vi "NMEA serial.vi"() -> ()   [LabVIEW 2016, in "AIRMAR WeatherCaster.lvlib"]
uses:
  AIRMAR WeatherCaster.lvlib
  NMEA_WIMDA-data.ctl
  NMEA_GPRMC-data.ctl
  NMEA_LatitudeDirection.ctl
  NMEA_LongitudeDirection.ctl
  <vilib>/Utility/miscctls.llb/LVPointTypeDef.ctl
  <vilib>/Instr/_visa.llb/VISA Configure Serial Port (Instr).vi
panel:
  out "$GPRMC-message_OUT":T1={"TimeStamp"=timestamp(0 s since 1904-01-01), "Validity"=FALSE, "Latitude"=0.0, "Latitude-Direction"=enum."North", "Longitude"=0.0, "Longitude-Direction"=enum."East", "Speed in knots"=0.0, "True course"=0.0, "Date Stamp"=timestamp(0 s since 1904-01-01), "Magnetic Variation (East/West)"=0.0} {"Magnetic Variation (East/West)" format="%.02f [deg]"; "Date Stamp" format="%<%x>T"; "True course" format="%.02f [deg]"; "Speed in knots" format="%.02f [kts]"; "Longitude" format="%0.4f [long]"; "Latitude" format="%.04f [lat]"; "TimeStamp" format="%<%.2X>T"}
  out "风向_真角":dbl caption="风向"
  out "风速_m/s":dbl caption="风速"
  out "风速_节":dbl caption="风速"
  out "气温_摄氏度":dbl caption="气温"
  out "气压_bars":dbl caption="气压"
  out "气压_英寸汞柱":dbl caption="气压"
  out "匹配语句":string
  out "$WIMDA-message_OUT":T4
  in  "串口打开":bool
  out "RAW DATA":string
  in  "baud rate (9600)":u32(ring)=4800 caption="波特率" items=["1200"=1200, "2400"=2400, "4800"=4800, "9600"=9600, "38400"=38400, "115200"=115200]
  in  "VISA resource name":refnum<visa-resource-name> caption="串口"
  # "°"
  # "m/s"
  # "节"
  # "℃"
  # "bars"
  # "英寸汞柱"
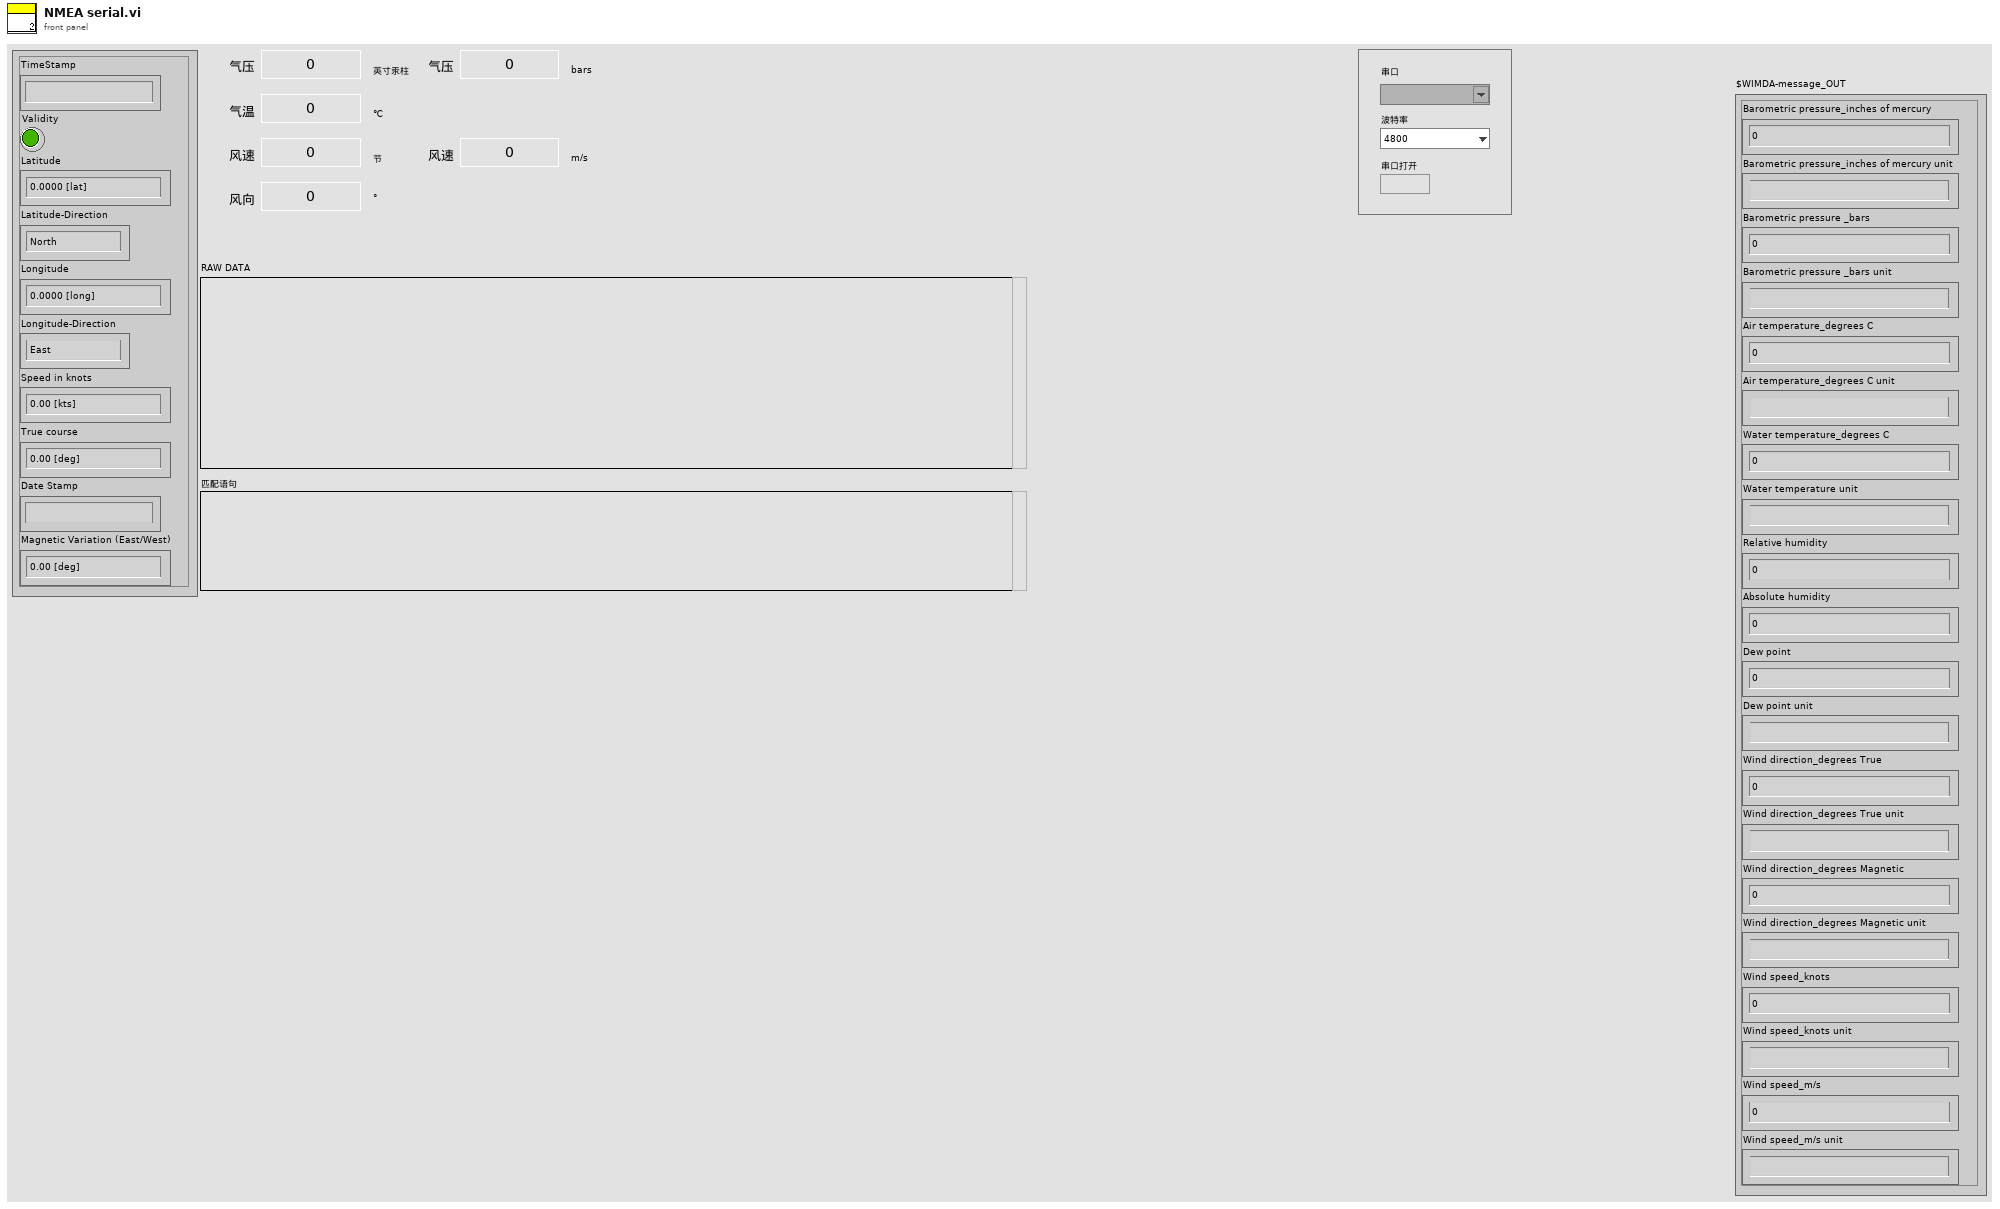
[diagram p1: front panel]
types:
  T1 = typedef "AIRMAR WeatherCaster.lvlib/NMEA_GPRMC-data.ctl" = cluster{"TimeStamp":timestamp, "Validity":bool, "Latitude":dbl, "Latitude-Direction":T2, "Longitude":dbl, "Longitude-Direction":T3, "Speed in knots":dbl, "True course":dbl, "Date Stamp":timestamp, "Magnetic Variation (East/West)":dbl}
  T2 = typedef "AIRMAR WeatherCaster.lvlib/NMEA_LatitudeDirection.ctl" = enum16{"", "North", "South"}
  T3 = typedef "AIRMAR WeatherCaster.lvlib/NMEA_LongitudeDirection.ctl" = enum16{"", "East", "West"}
  T4 = typedef "AIRMAR WeatherCaster.lvlib/NMEA_WIMDA-data.ctl" = cluster{"Barometric pressure_inches of mercury":dbl, "Barometric pressure_inches of mercury unit":string, "Barometric pressure _bars":dbl, "Barometric pressure _bars unit":string, "Air temperature_degrees C":dbl, "Air temperature_degrees C unit":string, "Water temperature_degrees C":dbl, "Water temperature unit":string, "Relative humidity":dbl, "Absolute humidity":dbl, "Dew point":dbl, "Dew point unit":string, "Wind direction_degrees True":dbl, "Wind direction_degrees True unit":string, "Wind direction_degrees Magnetic":dbl, "Wind direction_degrees Magnetic unit":string, "Wind speed_knots":dbl, "Wind speed_knots unit":string, "Wind speed_m/s":dbl, "Wind speed_m/s unit":string}
  T5 = typedef "LVPointTypeDef.ctl" = cluster{"Horizontal":i16, "Vertical":i16}
  T6 = typedef "LVDateTimeRec.ctl" = cluster{"秒数的小数部分":dbl, "秒":i32, "分":i32, "时":i32, "日":i32, "月":i32, "年":i32, "天数（周）":i32, "天数（年）":i32, "DST":i32}
  T7 = enum8{"Enabled", "Disabled", "Disabled and Grayed Out"}
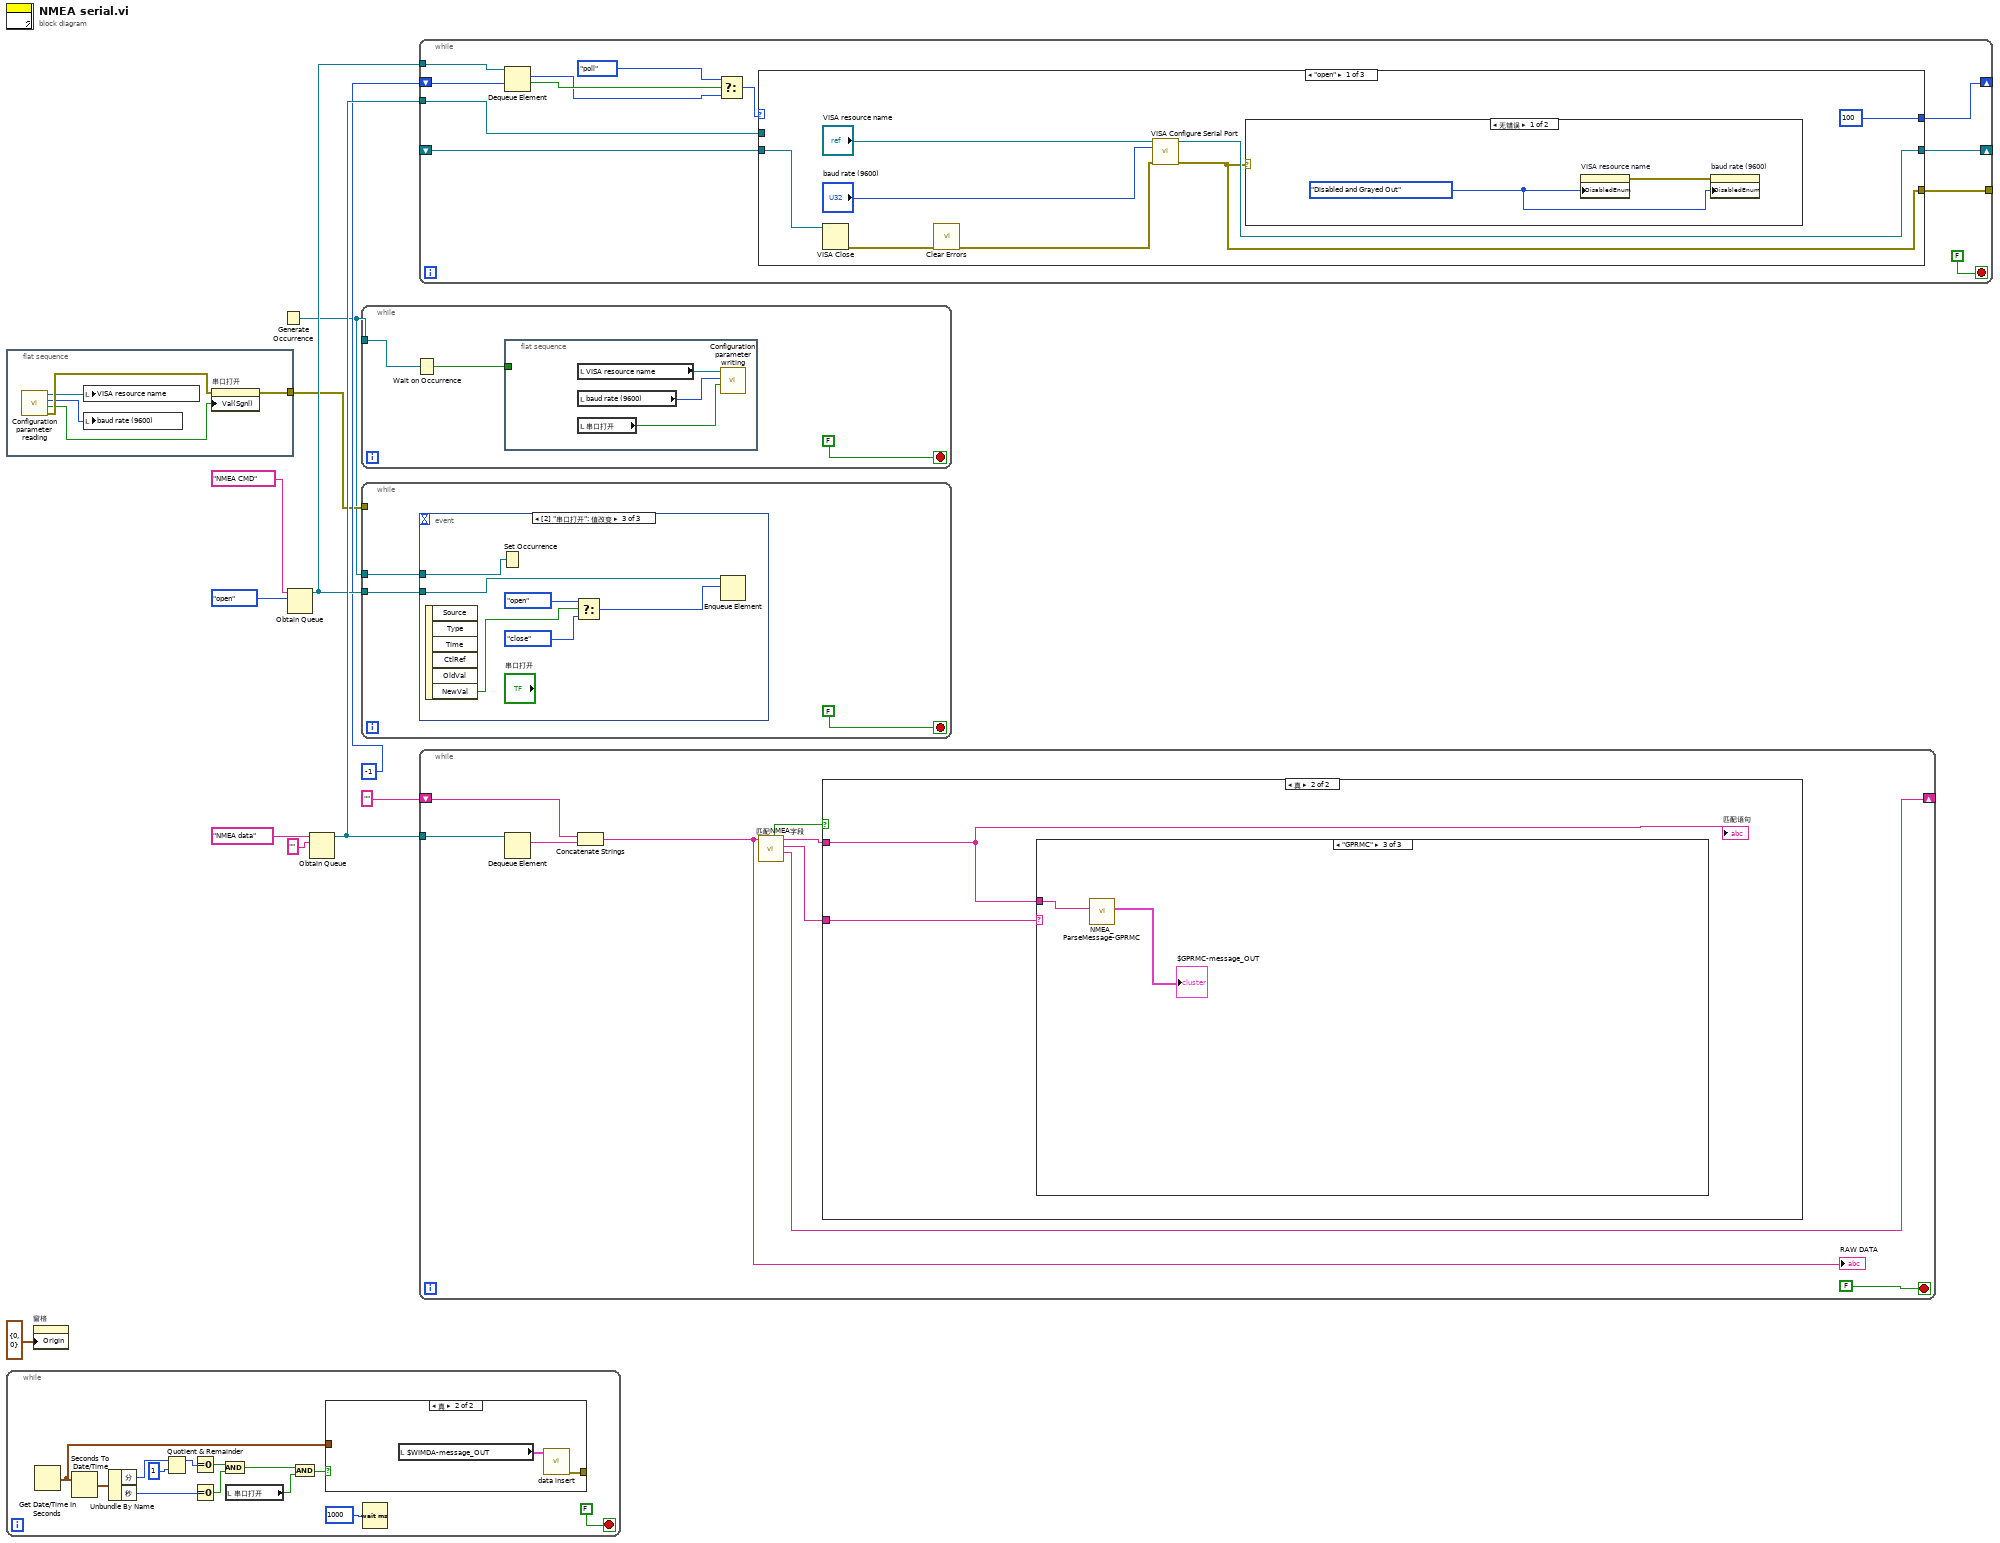
[diagram p0: block diagram]
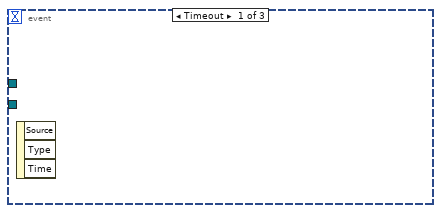
[diagram p3: hidden frame]
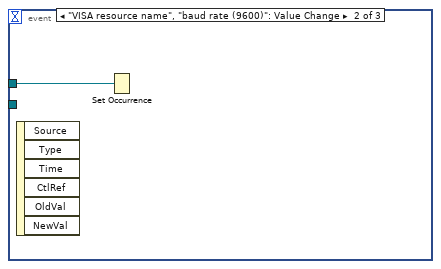
[diagram p4: hidden frame]
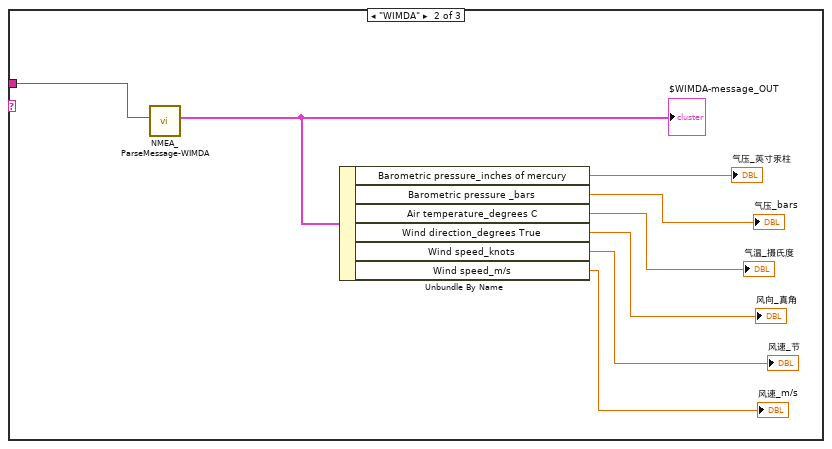
[diagram p7: hidden frame]
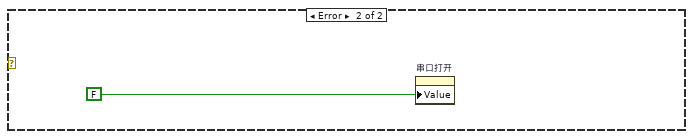
[diagram p8: hidden frame]
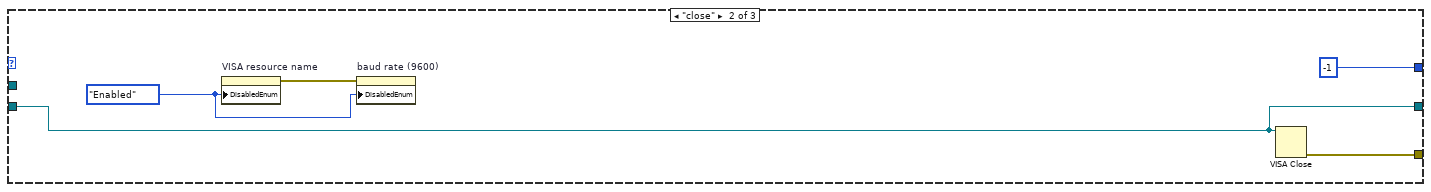
[diagram p9: hidden frame]
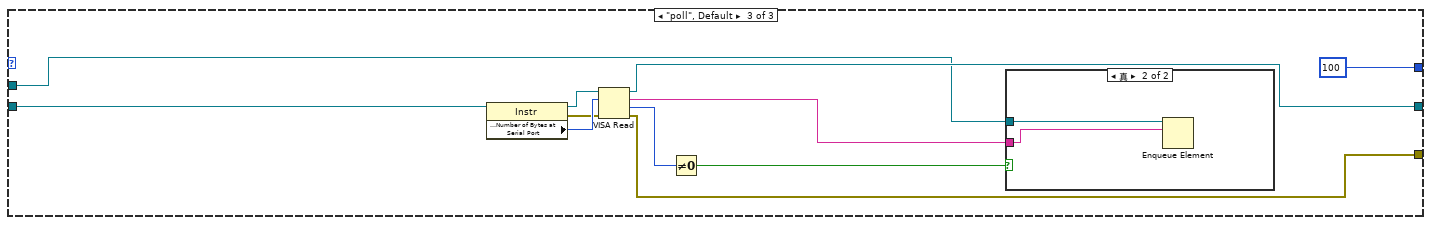
[diagram p10: hidden frame]
diagram:
  n1 = flat-sequence {
    tunnel: [w16] -> w2
    frame #0 {
      n2 = call "Configuration parameter reading.vi"() -> ("error out"=w15:errorcluster, "enable"=w12:bool, "baud rate (9600)"=w14:u32, "VISA resource name"=w13:refnum<visa-resource-name>)  [unwired: 8 in]
      n3 = local write "VISA resource name"(w13) -> ()
      n4 = local write "baud rate (9600)"(w14) -> ()
      n5 = property on="串口打开" class="Bool (严格)"(error in=w15, "Val(Sgnl)"=w12) -> (error out=w16:errorcluster)  [unwired: 1 in, 1 out]
    }
  }
  n6 = while {
    stop <- FALSE stop-if-true
    n7 = Get Date/Time In Seconds() -> (seconds since 1Jan1904=w20:timestamp)
    n8 = Seconds To Date/Time(time stamp (now)=w20) -> (date time rec=w28:T6)  [unwired: 1 in]
    n9 = Unbundle By Name(w28) -> ("分"=w27:i32, "秒"=w24:i32)
    n10 = Quotient & Remainder(x=w27, y=1) -> (x-y*floor(x/y)=w25:i32)  [unwired: 1 out]
    n11 = Equal To 0?(x=w25) -> (x = 0?=w23:bool)
    n12 = Equal To 0?(x=w24) -> (x = 0?=w22:bool)
    n13 = And(x=w23, y=w22) -> (x .and. y?=w21:bool)
    n14 = local read "串口打开"() -> (w17:bool)
    n15 = And(x=w21, y=w17) -> (x .and. y?=w18:bool)
    n16 = case shown="真" w18 {
      tunnel: w20 -> [_ _]
      tunnel: [_ w30] -> _
      frame False {
      }
      frame True {
        n17 = local read "$WIMDA-message_OUT"() -> (w31:T4)
        n18 = call "data insert.vi"("WIMDA-data"=w31) -> ("error out"=w30:errorcluster)  [unwired: 10 in]
      }
    }
    n19 = Wait (ms)(milliseconds to wait=u32 1000 ("等待时间（毫秒）")) -> ()  [unwired: 1 out]
  }
  n20 = property on="窗格" class="Pane"("Origin"=T5 {"Horizontal"=0, "Vertical"=0} ("原点")) -> ()  [unwired: 2 in, 2 out]
  n21 = Generate Occurrence() -> (w1:refnum<k4>)
  n22 = Obtain Queue(name (unnamed)="NMEA CMD" ("名称（未命名）"), element data type=enum16{"open", "close", "poll"}."open" ("枚举")) -> (queue out=w5:refnum<queue>)  [unwired: 3 in, 2 out]
  n23 = Obtain Queue(name (unnamed)="NMEA data" ("名称（未命名）"), element data type="") -> (queue out=w7:refnum<queue>)  [unwired: 3 in, 2 out]
  n24 = while {
    tunnel: w1 -> [w33]
    stop <- FALSE stop-if-true
    n25 = Wait on Occurrence(2:w33) -> (0:w32:bool)  [unwired: 2 in]
    n26 = flat-sequence {
      tunnel: w32 -> [_]
      frame #0 {
        n27 = local read "VISA resource name"() -> (w37:refnum<visa-resource-name>)
        n28 = local read "baud rate (9600)"() -> (w36:u32)
        n29 = local read "串口打开"() -> (w35:bool)
        n30 = call "Configuration parameter writing.vi"("enable"=w35, "baud rate (9600)"=w36, "VISA resource name"=w37) -> ()  [unwired: 9 in]
      }
    }
  }
  n31 = while {
    tunnel: w5 -> [w39]
    tunnel: w2 -> [_]
    tunnel: w1 -> [w38]
    stop <- FALSE stop-if-true
    n32 = event shown="[2] \"串口打开\": 值改变" {
      selector: _ -> [_ _ _]
      dyn-events: _ -> [_ _ _]
      timeout: _ -> [_ _ _]
      tunnel: w39 -> [_ _ w47]
      tunnel: w38 -> [_ w41 w42]
      event Timeout {
        n33 = event-data() -> ()  [unwired: 1 in, 3 out]
      }
      event "VISA resource name", "baud rate (9600)": Value Change {
        n34 = event-data() -> ()  [unwired: 1 in, 6 out]
        n35 = Set Occurrence(w41) -> ()
      }
      event "串口打开": Value Change {
        n36 = event-data() -> ("NewVal"=w46:bool)  [unwired: 1 in, 5 out]
        n37 = Set Occurrence(w42) -> ()
        n38 = Select(t=enum16{"open", "close", "poll"}."open" ("元素"), s=w46, f=enum16{"open", "close", "poll"}."close") -> (s? t:f=w44:enum16{"open", "close", "poll"})
        n39 = Enqueue Element(queue=w47, element=w44) -> ()  [unwired: 2 in, 3 out]
      }
    }
  }
  n40 = while {
    shift-right: [w59] -> _
    shift-left: _ -> [w58]
    tunnel: w5 -> [w57]
    tunnel: [w56] -> _
    tunnel: w7 -> [w55]
    shift-right: [w48] -> _
    shift-left: -1 ("超时毫秒(-1)") -> [w49]
    stop <- FALSE stop-if-true
    n41 = Dequeue Element(queue=w57, timeout in ms (-1)=w49) -> (element=w51:enum16{"open", "close", "poll"}, timed out?=w53:bool)  [unwired: 1 in, 2 out]
    n42 = Select(t=enum16{"open", "close", "poll"}."poll" ("枚举"), s=w53, f=w51) -> (s? t:f=w50:enum16{"open", "close", "poll"})
    n43 = case shown="\"open\"" w50 {
      tunnel: [w65 w75 w86] -> w59
      tunnel: w58 -> [w64 w75 w84]
      tunnel: [w60 w74 w85] -> w56
      tunnel: w55 -> [_ _ w81]
      tunnel: [100 ("超时毫秒(-1)") -1 ("超时毫秒(-1)") 100 ("超时毫秒(-1)")] -> w48
      frame "open" {
        n44 = VISA Close(VISA resource name=w64) -> (error out=w63:errorcluster)  [unwired: 1 in]
        n45 = call <vilib>:"Clear Errors.vi"("error in (no error)"=w63) -> ("error out"=w62:errorcluster)  [unwired: 5 in, 1 out]
        n46 = call-poly "VISA Configure Serial Port"("VISA resource name"="VISA resource name", "baud rate (9600)"="baud rate (9600)", "error in (no error)"=w62) -> ("VISA resource name out"=w65:refnum<visa-resource-name>, "error out"=w60:errorcluster)  [unwired: 11 in]
        n47 = case shown="无错误" w60 {
          frame No Error {
            w69 = T7."Disabled and Grayed Out" ("禁用")
            n48 = property on="VISA resource name" class="VISAName"("DisabledEnum"=w69) -> (error out=w68:errorcluster)  [unwired: 2 in, 1 out]
            n49 = property on="baud rate (9600)" class="Ring (严格)"(error in=w68, "DisabledEnum"=w69) -> ()  [unwired: 1 in, 2 out]
          }
          frame Error {
            n50 = property on="串口打开" class="Bool (严格)"("Value"=FALSE ("串口打开")) -> ()  [unwired: 2 in, 2 out]
          }
        }
      }
      frame "close" {
        w71 = T7."Enabled" ("禁用")
        n51 = property on="VISA resource name" class="VISAName"("DisabledEnum"=w71) -> (error out=w72:errorcluster)  [unwired: 2 in, 1 out]
        n52 = property on="baud rate (9600)" class="Ring (严格)"(error in=w72, "DisabledEnum"=w71) -> ()  [unwired: 1 in, 2 out]
        n53 = VISA Close(VISA resource name=w75) -> (error out=w74:errorcluster)  [unwired: 1 in]
      }
      frame "poll", Default {
        n54 = property class="Instr"(reference=w84) -> (reference out=w83:refnum<visa-resource-name>, error out=w77:errorcluster, "Serial Settings:Number of Bytes at Serial Port"=w82:u32)  [unwired: 1 in]
        n55 = VISA Read(VISA resource name=w83, byte count=w82, error in (no error)=w77) -> (VISA resource name out=w86:refnum<visa-resource-name>, read buffer=w80:string, return count=w79:u32, error out=w85:errorcluster)
        n56 = Not Equal To 0?(x=w79) -> (x != 0?=w78:bool)
        n57 = case shown="真" w78 {
          tunnel: w81 -> [_ w88]
          tunnel: w80 -> [_ w87]
          frame False {
          }
          frame True {
            n58 = Enqueue Element(queue=w88, element=w87) -> ()  [unwired: 2 in, 3 out]
          }
        }
      }
    }
  }
  n59 = while {
    tunnel: w7 -> [w97]
    shift-right: [w90] -> _
    shift-left: "" -> [w95]
    stop <- FALSE stop-if-true
    n60 = Dequeue Element(queue=w97) -> (element=w96:string)  [unwired: 2 in, 3 out]
    n61 = Concatenate Strings(w95, w96) -> (w93:string)
    "RAW DATA" <- w93
    n62 = call "匹配NMEA字段.vi"("输入字符串"=w93) -> ("未匹配语句"=w90:string, "NMEA语句"=w89:string, "匹配语句"=w92:string, "匹配"=w91:bool)  [unwired: 7 in]
    n63 = case shown="真" w91 {
      tunnel: w92 -> [_ w99]
      tunnel: w89 -> [_ w98]
      frame False {
      }
      frame True {
        n64 = case shown="\"GPRMC\"" w98 {
          tunnel: w99 -> [_ w107 w109]
          frame "假", Default {
          }
          frame "WIMDA" {
            n65 = call "NMEA_ParseMessage-WIMDA.vi"("$WIMDA-message_IN"=w107) -> ("$WIMDA-message_OUT"=w106:T4)  [unwired: 9 in, 1 out]
            "$WIMDA-message_OUT" <- w106
            n66 = Unbundle By Name(w106) -> ("Barometric pressure_inches of mercury"=→"气压_英寸汞柱":dbl, "Barometric pressure _bars"=→"气压_bars":dbl, "Air temperature_degrees C"=→"气温_摄氏度":dbl, "Wind direction_degrees True"=→"风向_真角":dbl, "Wind speed_knots"=→"风速_节":dbl, "Wind speed_m/s"=→"风速_m/s":dbl)
          }
          frame "GPRMC" {
            n67 = call "NMEA_ParseMessage-GPRMC.vi"("$GPRMC-message_IN"=w109) -> ("$GPRMC-message_OUT"=→"$GPRMC-message_OUT":T1)  [unwired: 9 in, 1 out]
          }
        }
        "匹配语句" <- w99
      }
    }
  }
